vi "Pre-Install Custom Action.vi"(10 "Variant":variant) -> (0 "Error Out":errorcluster)   [LabVIEW 2011]
uses:
  <vilib>/registry/registry.llb/Registry SAM.ctl
  <vilib>/LabVIEW Hacker/LVH-Toolbox/Common/LVH-Common.lvlib
panel:
  in  "Status":string
  out "Slide":u8(slide) scale=0.0..100.0
  in  "Cancel Button":bool
  in  "Install Adept Runtime":bool
  in  "Install VC++":bool
  in  "Adept Installed":bool
  in  "VC++ Installed":bool
  in  "Adept":bool caption="Blank Button"
  in  "VC++":bool caption="Blank Button"
  # "In order to use the Adept LabVIEW Interface the VC++ 2012 Redistributable and the \nAdept Runtime must be installed.  Please install the missing components below."
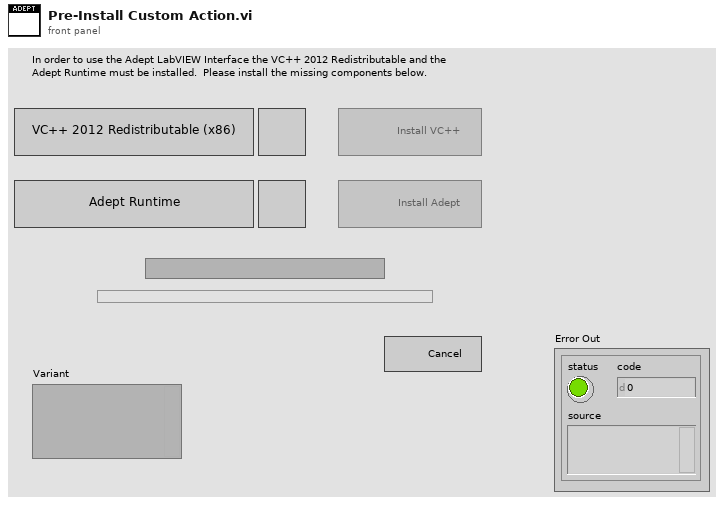
[diagram p1: front panel]
types:
  T1 = typedef "Registry SAM.ctl" = enum32{"KEY_QUERY_VALUE", "KEY_SET_VALUE", "KEY_CREATE_SUB_KEY", "KEY_ENUMERATE_SUB_KEYS", "KEY_NOTIFY", "KEY_CREATE_LINK", "KEY_READ", "KEY_WRITE", "KEY_ALL_ACCESS", "KEY_READ | KEY_WRITE"}
  T2 = enum8{"Enabled", "Disabled", "Disabled and Grayed Out"}
  T3 = enum16{"open", "open or create", "create or replace", "create", "open (read only)"}
  T4 = typedef "Registry refnum.ctl" = refnum<k1>
  T5 = cluster{"numSubKeys":i32, "maxSubKeyLen":i32, "maxSubKeyClassLen":i32}
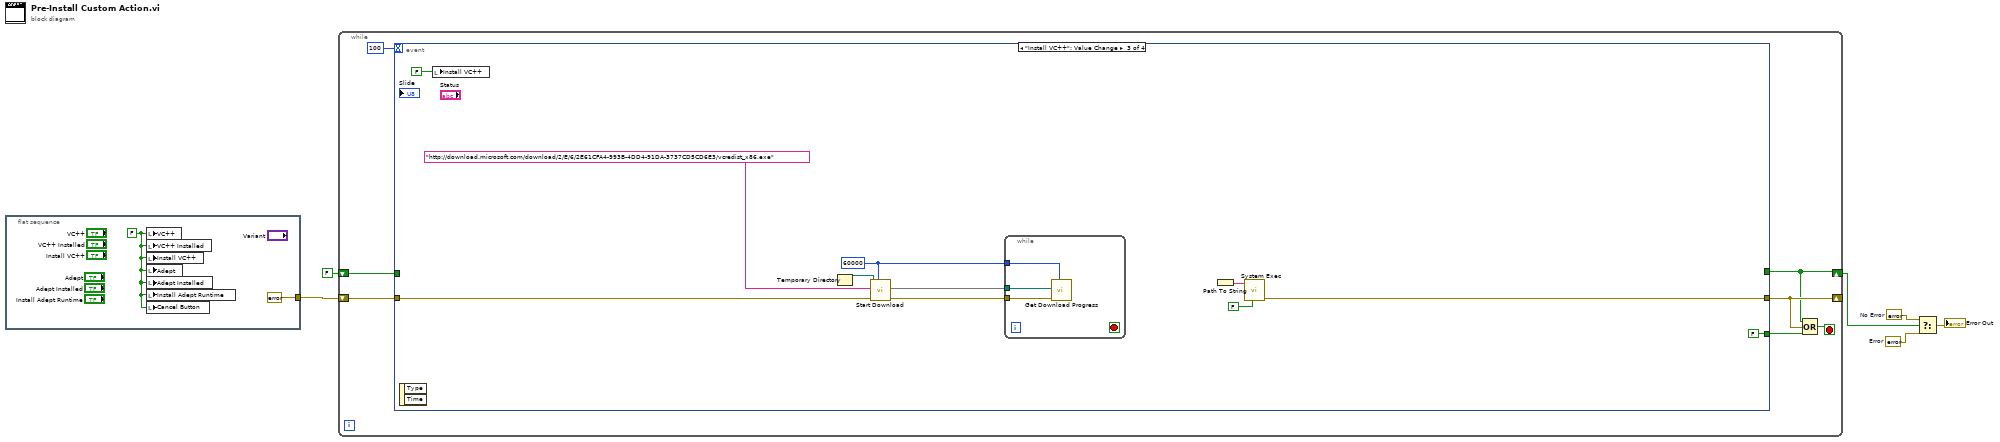
[diagram p0: block diagram]
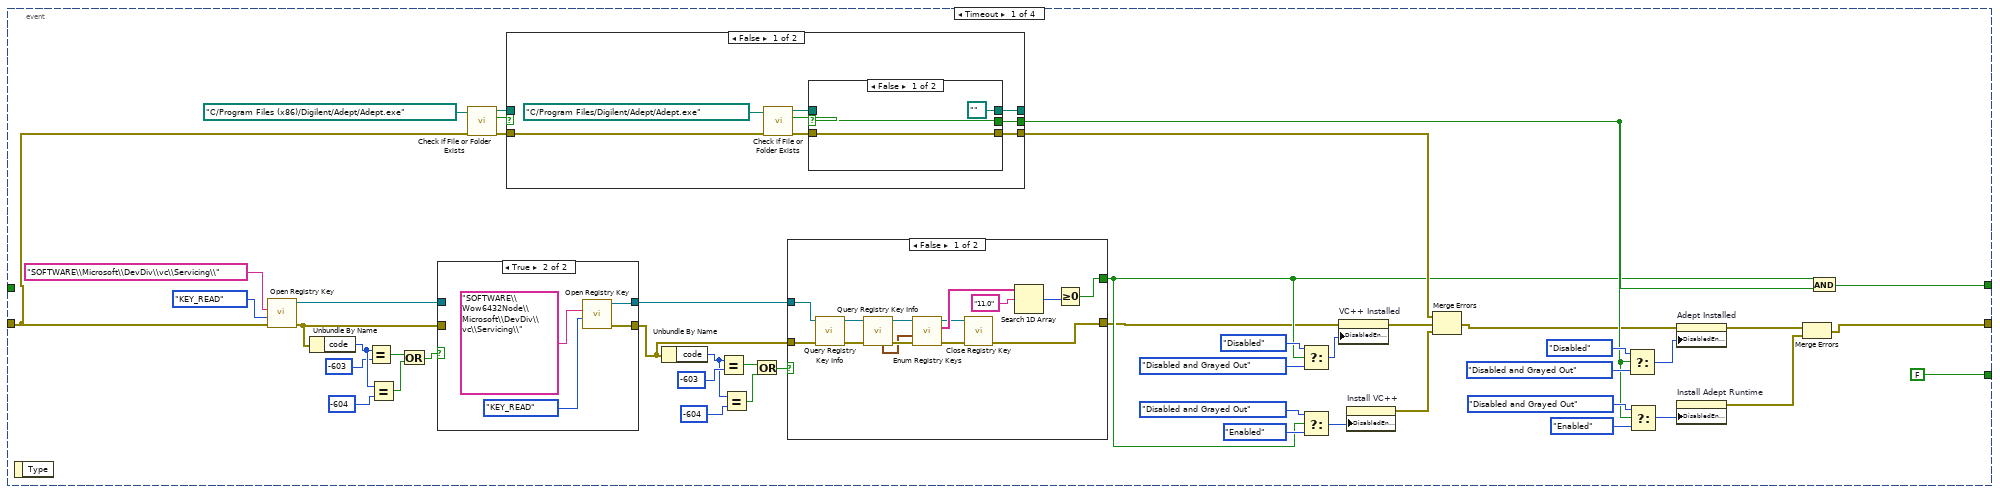
[diagram p2: hidden frame]
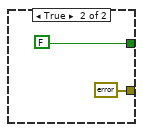
[diagram p3: hidden frame]
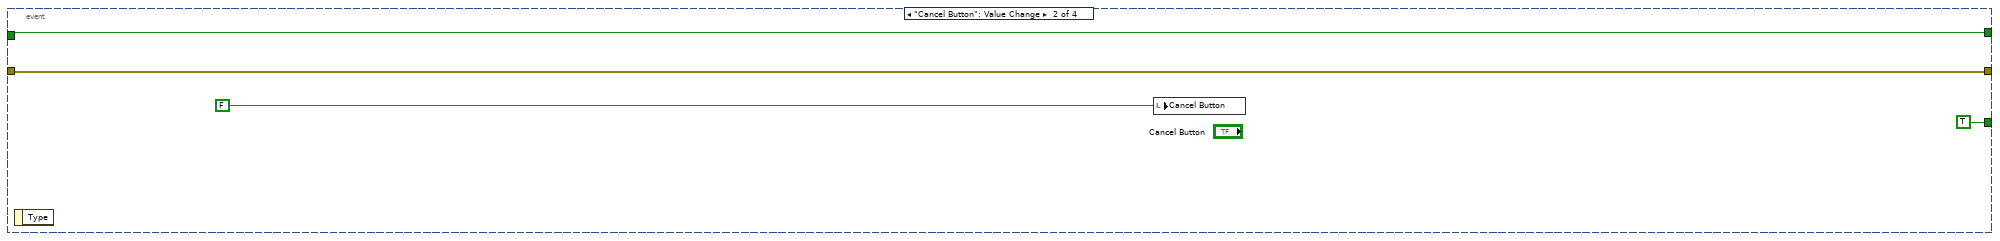
[diagram p7: hidden frame]
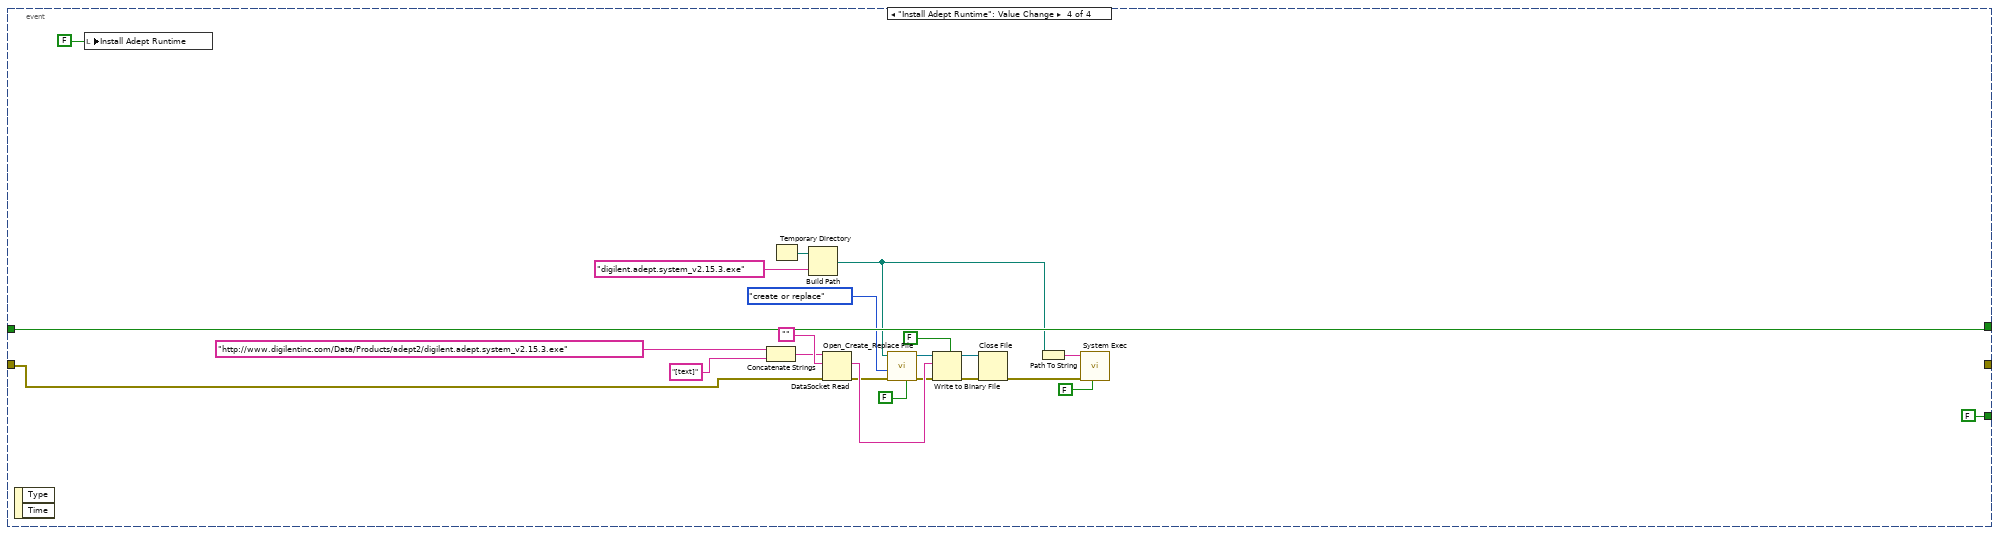
[diagram p8: hidden frame]
diagram:
  w3 = errorcluster {"status"=FALSE, "code"=0, "source"=""}  # No Error
  w2 = errorcluster {"status"=TRUE, "code"=5000, "source"="Adept Interface Pre Reqs Not Met"}  # Error
  n1 = flat-sequence {
    tunnel: [errorcluster {"status"=FALSE, "code"=0, "source"=""} ("Error In")] -> w6
    frame #0 {
      w8 = FALSE ("VC++")
      n2 = local write "VC++"(w8) -> ()
      n3 = local write "VC++ Installed"(w8) -> ()
      n4 = local write "Install VC++"(w8) -> ()
      n5 = local write "Adept"(w8) -> ()
      n6 = local write "Adept Installed"(w8) -> ()
      n7 = local write "Install Adept Runtime"(w8) -> ()
      n8 = local write "Cancel Button"(w8) -> ()
    }
  }
  n9 = while {
    shift-right: [w13] -> _
    shift-left: w6 -> [w15]
    shift-right: [w9] -> w4
    shift-left: FALSE -> [w11]
    stop <- w14 stop-if-true
    n10 = event shown="[2] \"Install VC++\": Value Change" {
      selector: _ -> [_ _ _ _]
      dyn-events: _ -> [_ _ _ _]
      timeout: 100 -> [_ _ _ _]
      tunnel: w15 -> [w29 w103 w109 w121]
      tunnel: [FALSE TRUE FALSE FALSE] -> w12
      tunnel: [w45 w103 w114 _] -> w13
      tunnel: w11 -> [_ w102 _ w141]
      tunnel: [w44 w102 _ w141] -> w9
      event Timeout {
        n11 = event-data() -> ()  [unwired: 1 in, 1 out]
        n12 = call <vilib>:"Open Registry Key.vi"("error in (no error)"=w29, "security access mask (KEY_READ | KEY_WRITE)"=Registry_SAM."KEY_READ", "subkey"="SOFTWARE\\Microsoft\\DevDiv\\vc\\Servicing\\") -> ("error out"=w36:errorcluster, "refnum out"=w37:T4)  [unwired: 7 in]
        n13 = Unbundle By Name(w36) -> ("code"=w41:i32)
        n14 = Equal?(x=w41, y=-603) -> (x = y?=w39:bool)
        n15 = Equal?(x=w41, y=-604) -> (x = y?=w42:bool)
        n16 = Or(x=w39, y=w42) -> (x .or. y?=w38:bool)
        n17 = case shown="True" w38 {
          tunnel: w36 -> [w96 _]
          tunnel: [w97 w100] -> w17
          tunnel: w37 -> [w97 _]
          tunnel: [w96 w99] -> w18
          frame False {
            # "Found x32 Entry"
          }
          frame True {
            n18 = call <vilib>:"Open Registry Key.vi"("security access mask (KEY_READ | KEY_WRITE)"=Registry_SAM."KEY_READ", "subkey"="SOFTWARE\\Wow6432Node\\Microsoft\\DevDiv\\vc\\Servicing\\") -> ("error out"=w99:errorcluster, "refnum out"=w100:T4)  [unwired: 8 in]
          }
        }
        n19 = call <vilib>:"Check if File or Folder Exists.vi"("error in (no error)"=w29, "path"=path "C:/Program Files (x86)/Digilent/Adept/Adept.exe") -> ("error out"=w30:errorcluster, "file or folder exists?"=w32:bool, "dup path"=w31:path)  [unwired: 7 in]
        n20 = case shown="False" w32 {
          selector: w32 -> [_ w93]
          tunnel: w31 -> [_ w95]
          tunnel: w30 -> [w85 w94]
          tunnel: [w84 w95] -> _
          tunnel: [w80 w94] -> w28
          tunnel: [w79 w93] -> w27
          frame False {
            n21 = call <vilib>:"Check if File or Folder Exists.vi"("error in (no error)"=w85, "path"=path "C:/Program Files/Digilent/Adept/Adept.exe") -> ("error out"=w81:errorcluster, "file or folder exists?"=w82:bool, "dup path"=w83:path)  [unwired: 7 in]
            n22 = case shown="False" w82 {
              selector: w82 -> [w88 w90]
              tunnel: [path "" ("dup path") w92] -> w84
              tunnel: w83 -> [_ w92]
              tunnel: w81 -> [w89 w91]
              tunnel: [w89 w91] -> w80
              tunnel: [w88 w90] -> w79
              frame False {
              }
              frame True {
              }
            }
          }
          frame True {
            # "Insalled under (x86)"
          }
        }
        n23 = Unbundle By Name(w18) -> ("code"=w22:i32)
        n24 = Equal?(x=w22, y=-603) -> (x = y?=w24:bool)
        n25 = Equal?(x=w22, y=-604) -> (x = y?=w21:bool)
        n26 = Or(x=w24, y=w21) -> (x .or. y?=w20:bool)
        n27 = case shown="False" w20 {
          tunnel: [w67 FALSE] -> w19
          tunnel: w18 -> [w66 _]
          tunnel: w17 -> [w65 _]
          tunnel: [w64 errorcluster {"status"=FALSE, "code"=0, "source"=""} ("error out")] -> w16
          frame False {
            n28 = call <vilib>:"Query Registry Key Info.vi"("error in (no error)"=w66, "refnum"=w65) -> ("error out"=w70:errorcluster, "refnum out"=w69:T4)  [unwired: 5 in, 3 out]
            n29 = call <vilib>:"Query Registry Key Info.vi"("error in (no error)"=w70, "refnum"=w69) -> ("error out"=w71:errorcluster, "refnum out"=w68:T4, "subkey info"=w63:T5)  [unwired: 5 in, 2 out]
            n30 = call <vilib>:"Enum Registry Keys.vi"("error in (no error)"=w71, "subkey info"=w63, "refnum"=w68) -> ("error out"=w73:errorcluster, "subkeys"=w74:string[], "refnum out"=w72:T4)  [unwired: 6 in]
            n31 = call <vilib>:"Close Registry Key.vi"("error in (no error)"=w73, "refnum"=w72) -> ("error out"=w64:errorcluster)  [unwired: 5 in]
            n32 = Search 1D Array(1D array=w74, element="11.0") -> (index of element=w76:i32)  [unwired: 1 in]
            n33 = Greater Or Equal To 0?(x=w76) -> (x >= 0?=w67:bool)
          }
          frame True {
          }
        }
        n34 = Select(t=T2."Disabled" ("Disabled"), s=w19, f=T2."Disabled and Grayed Out" ("Disabled")) -> (s? t:f=w46:T2)
        n35 = Select(t=T2."Disabled and Grayed Out" ("Disabled"), s=w19, f=T2."Enabled" ("Disabled")) -> (s? t:f=w54:T2)
        n36 = property on="VC++ Installed" class="Bool (strict)"(error in=w16, "DisabledEnum"=w46) -> (error out=w55:errorcluster)  [unwired: 1 in, 1 out]
        n37 = property on="Install VC++" class="Bool (strict)"("DisabledEnum"=w54) -> (error out=w56:errorcluster)  [unwired: 2 in, 1 out]
        n38 = Merge Errors(w28, w55, w56) -> (w26:errorcluster)
        n39 = Select(t=T2."Disabled" ("Disabled"), s=w27, f=T2."Disabled and Grayed Out" ("Disabled")) -> (s? t:f=w50:T2)
        n40 = Select(t=T2."Disabled and Grayed Out" ("Disabled"), s=w27, f=T2."Enabled" ("Disabled")) -> (s? t:f=w59:T2)
        n41 = property on="Adept Installed" class="Bool (strict)"(error in=w26, "DisabledEnum"=w50) -> (error out=w60:errorcluster)  [unwired: 1 in, 1 out]
        n42 = property on="Install Adept Runtime" class="Bool (strict)"("DisabledEnum"=w59) -> (error out=w61:errorcluster)  [unwired: 2 in, 1 out]
        n43 = Merge Errors(w60, w61) -> (w45:errorcluster)
        n44 = And(x=w19, y=w27) -> (x .and. y?=w44:bool)
      }
      event "Cancel Button": Value Change {
        n45 = event-data() -> ()  [unwired: 1 in, 1 out]
        n46 = local write "Cancel Button"(FALSE ("Cancel Button")) -> ()
      }
      event "Install VC++": Value Change {
        w106 = 60000 ("Timeout (ms)")
        n47 = event-data() -> ()  [unwired: 1 in, 2 out]
        n48 = local write "Install VC++"(FALSE ("Install VC++")) -> ()
        n49 = Temporary Directory() -> (w108:path)
        n50 = call <vilib>:"Start Download.vi"(7:w106, "Error In"=w109, "Download Directory"="http://download.microsoft.com/download/2/E/6/2E61CFA4-993B-4DD4-91DA-3737CD5CD6E3/vcredist_x86.exe" ("URL of PDF:"), "URL"=w108) -> ("Error Out"=w111:errorcluster, 2:w110)  [unwired: 5 in, 1 out]
        n51 = while {
          tunnel: w111 -> [w119]
          tunnel: w110 -> [w118]
          tunnel: w106 -> [w117]
          stop <- _ stop-if-true
          n52 = call <vilib>:"Get Download Progress.vi"("Download Timeout (S)"=w117, "Error In"=w119, 10:w118) -> ()  [unwired: 4 in, 5 out]
        }
        n53 = Path To String() -> (string=w112:string)  [unwired: 1 in]
        n54 = call <vilib>:"System Exec.vi"("run minimized? (F)"=FALSE, "command line"=w112) -> ("error out"=w114:errorcluster)  [unwired: 6 in, 3 out]
      }
      event "Install Adept Runtime": Value Change {
        n55 = event-data() -> ()  [unwired: 1 in, 2 out]
        n56 = local write "Install Adept Runtime"(FALSE ("Install Adept Runtime")) -> ()
        n57 = Concatenate Strings("http://www.digilentinc.com/Data/Products/adept2/digilent.adept.system_v2.15.3.exe", "[text]" ("string")) -> (w133:string)
        n58 = Temporary Directory() -> (w127:path)
        n59 = Build Path(base path=w127, name or relative path="digilent.adept.system_v2.15.3.exe") -> (appended path=w123:path)
        n60 = DataSocket Read(8:w121, 10:"", 11:w133) -> (0:w132:errorcluster, 2:w139:string)  [unwired: 2 in, 5 out]
        n61 = call <vilib>:"Open_Create_Replace File.vi"("advisory dialog? (display:T)"=FALSE, "error in (no error)"=w132, "function (open:0)"=T3."create or replace", "file path"=w123) -> ("error out"=w131:errorcluster, "refnum"=w130:refnum<file>)  [unwired: 4 in, 2 out]
        n62 = Write to Binary File(file (use dialog)=w130, data=w139, error in=w131, 5:FALSE ("prepend array or string size? (T)")) -> (refnum out=w138:refnum<file>, error out=w137:errorcluster)  [unwired: 2 in, 1 out]
        n63 = Close File(refnum=w138, error in=w137) -> (error out=w125:errorcluster)  [unwired: 1 out]
        n64 = Path To String(path=w123) -> (string=w122:string)
        n65 = call <vilib>:"System Exec.vi"("run minimized? (F)"=FALSE, "error in (no error)"=w125, "command line"=w122) -> ()  [unwired: 5 in, 4 out]
      }
    }
    n66 = Compound Arithmetic op=OR(w9, w13, w12) -> (w14:bool)
  }
  n67 = Select(t=w3, s=w4, f=w2) -> (s? t:f=→"Error Out":errorcluster)
